vi "Cal single extension given force.vi"() -> ()   [LabVIEW 2014]
panel:
  in  "Tab Control":enum32{"Page 1", "Page 2", "Page 3"}(tab)
  out "XY Graph":cluster{dbl[], dbl[]}[](graph)
  out "XY Graph 2":cluster{dbl[], dbl[]}(graph)
  out "XY Graph 3":cluster{dbl[], dbl[]}(graph)
  out "diff for phi29 rep (nm)":dbl[](array[numeric])
  out "diff for bind on ssDNA (nm)":dbl[](array[numeric])
  out "diff for bind on dsDNA (nm)":dbl[](array[numeric])
  out "Force Array (pN)":dbl[](array[numeric])
  in  "dF (pN)":dbl=0.05
  in  "End (pN)":dbl=50.0
  in  "Start (pN)":dbl=0.1
  in  "K for m51 bound (pN)":dbl=3500.0
  out "Extension (nm)":dbl
  out "expected contour length for dsDNA (nm)":dbl
  out "expected contour length for ssDNA (nm) 2":dbl
  # "3 nt or bp"
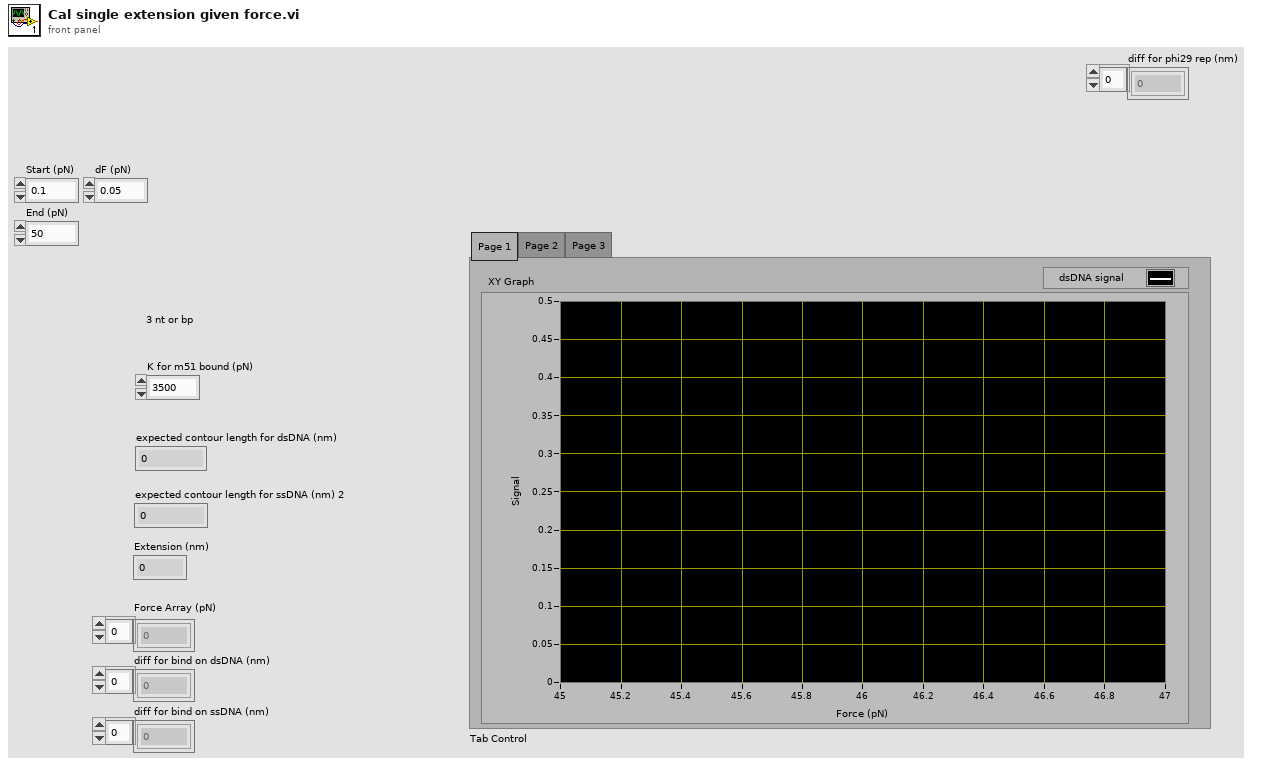
[diagram p1: front panel]
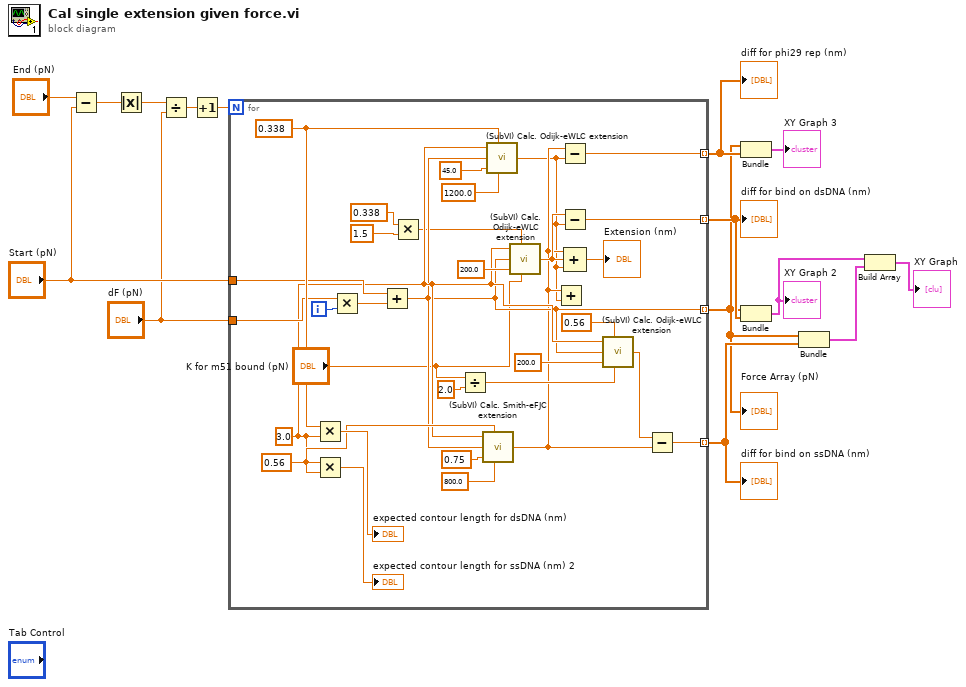
[diagram p0: block diagram]
diagram:
  n1 = Subtract(x="End (pN)", y="Start (pN)") -> (x-y=w13:dbl)
  n2 = Absolute Value(x=w13) -> (abs(x)=w12:dbl)
  n3 = Divide(x=w12, y="dF (pN)") -> (x/y=w10:dbl)
  n4 = Increment(x=w10) -> (x+1=w9:dbl)
  n5 = for {
    N: w9 -> [_]
    tunnel: [w36] -> w7 mode=indexing
    tunnel: [w34] -> w8 mode=indexing
    tunnel: "Start (pN)" -> [w30]
    tunnel: "dF (pN)" -> [w32]
    tunnel: [w25] -> w2 mode=indexing
    tunnel: [w17] -> w3 mode=indexing
    i -> [w33]
    w26 = 3.0 ("m51 bind nt")
    w46 = 0.338 ("nm/bp")
    w44 = 0.56 ("nm/nt")
    n6 = Multiply(x=w46, y=w26) -> (x*y=→"expected contour length for dsDNA (nm)":dbl)
    n7 = Multiply(x=w44, y=w26) -> (x*y=→"expected contour length for ssDNA (nm) 2":dbl)
    n8 = Multiply(x=w32, y=w33) -> (x*y=w31:dbl)
    n9 = Add(x=w30, y=w31) -> (x+y=w25:dbl)
    n10 = Multiply(x=0.338 ("nm/bp"), y=1.5 ("nm/bp")) -> (x*y=w16:dbl)
    n11 = Divide(x="K for m51 bound (pN)", y=2.0 ("Persistence length (nm)")) -> (x/y=w23:dbl)
    n12 = call "(SubVI) Calc. Smith-eFJC extension.vi"("ssDNA Length (nt)"=w26, "nm/nt"=w44, "Force (pN)"=w25, "Persistence length (nm)"=0.75, "Elastic modulus (pN)"=800.0) -> ("Extension (nm)"=w19:dbl)  [unwired: 2 in]
    n13 = call "(SubVI) Calc. Odijk-eWLC extension.vi"("dsDNA Length (bp)"=w26, "nm/bp"=w46, "Force (pN)"=w25, "Persistence length (nm)"=45.0, "Elastic modulus (pN)"=1200.0) -> ("Extension (nm)"=w18:dbl)  [unwired: 2 in]
    n14 = call "(SubVI) Calc. Odijk-eWLC extension.vi"("dsDNA Length (bp)"=w26, "nm/bp"=w16, "Force (pN)"=w25, "Persistence length (nm)"=200.0, "Elastic modulus (pN)"="K for m51 bound (pN)") -> ("Extension (nm)"=w35:dbl)  [unwired: 2 in]
    n15 = Add(x=w19, y=w18) -> ()  [unwired: 1 out]
    n16 = Subtract(x=w19, y=w18) -> (x-y=w17:dbl)
    n17 = Subtract(x=w35, y=w18) -> (x-y=w34:dbl)
    n18 = Compound Arithmetic op=ADD(w19, w35, w18) -> (→"Extension (nm)":dbl)
    n19 = call "(SubVI) Calc. Odijk-eWLC extension.vi"("dsDNA Length (bp)"=w26, "nm/bp"=0.56, "Force (pN)"=w25, "Persistence length (nm)"=200.0, "Elastic modulus (pN)"=w23) -> ("Extension (nm)"=w20:dbl)  [unwired: 2 in]
    n20 = Subtract(x=w20, y=w19) -> (x-y=w36:dbl)
  }
  "Force Array (pN)" <- w2
  "diff for bind on dsDNA (nm)" <- w8
  "diff for bind on ssDNA (nm)" <- w7
  "diff for phi29 rep (nm)" <- w3
  n21 = Bundle(w2, w3) -> (→"XY Graph 3":cluster{dbl[], dbl[]})  [unwired: 1 in]
  n22 = Bundle(w2, w8) -> (w4:cluster{dbl[], dbl[]})  [unwired: 1 in]
  "XY Graph 2" <- w4
  n23 = Bundle(w2, w7) -> (w6:cluster{dbl[], dbl[]})  [unwired: 1 in]
  n24 = Build Array(w4, w6) -> (→"XY Graph":cluster{dbl[], dbl[]}[])
